vi "PCO_CamLinkSetImageParameters.vi"(8 "error in (no error)":errorcluster {"code" format="%x"}, 9 "wYres":u16, 10 "wXres":u16, 11 "ph":u64) -> (0 "error out":errorcluster {"code" format="%x"}, 2 "ErrorMessage":i32 format="%x", 3 "ph out":u64)   [LabVIEW 2019, in "SDK.lvlib" / "SpecialCommandsEdge.lvlib"]
doc: "Sets the parameters for an image transfer. Required for CameraLink interface, and recommended for other interface types. Call this function when there is a change in the effective image size through ROI os binning, or switching to RAM segment (cameras with internal memory) where the image size differs from the current segment."
uses:
  SpecialCommandsEdge.lvlib
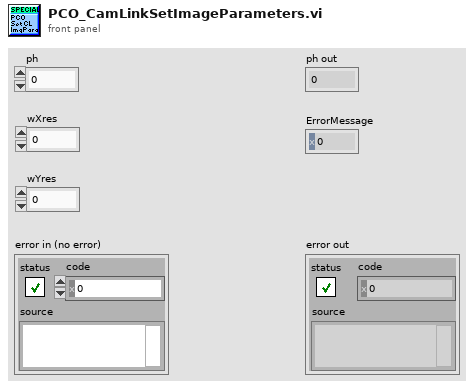
[diagram p1: front panel]
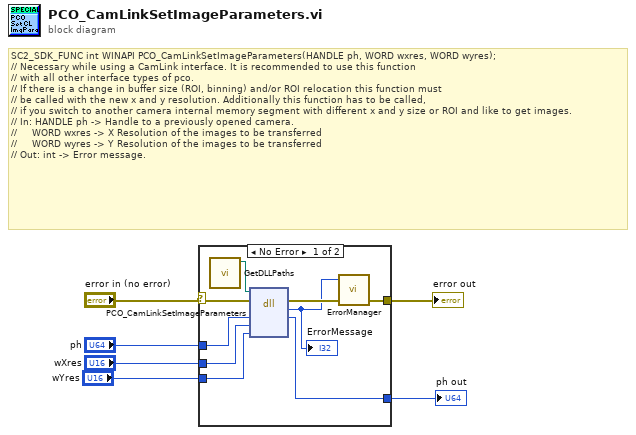
[diagram p0: block diagram]
diagram:
  # "SC2_SDK_FUNC int WINAPI PCO_CamLinkSetImageParameters(HANDLE ph, WORD wxres, WORD wyres);\n// Necessary while using a CamLink interface. It is recommended to use this function\n// with all other interface types of pco.\n// If there is a change in buffer size (ROI, binning) and/or ROI relocation this function must\n// be called with the new x and y resolution. Additionally this function has to be called,\n// if you switch to another camera internal memory segment with different x and y size or ROI and like to get images.\n// In: HANDLE ph -> Handle to a previously opened camera.\n//     WORD wxres -> X Resolution of the images to be transferred\n//     WORD wyres -> Y Resolution of the images to be transferred\n// Out: int -> Error message."
  n1 = case shown="No Error" "error in (no error)" {
    selector: "error in (no error)" -> [w13 w17]
    tunnel: "ph" -> [w15 w16]
    tunnel: [w14 w16] -> w5
    tunnel: [w11 w17] -> w4
    tunnel: "wXres" -> [w8 _]
    tunnel: "wYres" -> [w7 _]
    frame No Error {
      n2 = call "GetDLLPaths.vi"() -> ("SC2_Cam_Path"=w9:path)  [unwired: 8 in, 3 out]
      n3 = dll-call lib="?" fn="PCO_CamLinkSetImageParameters"(path in=w9, error in=w13, "ph"=w15, "wXres"=w8, "wYres"=w7) -> (error out=w12:errorcluster, "return type"=w10:i32, "ph"=w14:u64)  [unwired: 3 in, 1 out]
      "ErrorMessage" <- w10
      n4 = call "ErrorManager.vi"("error in (no error)"=w12, "error code"=w10) -> ("error out"=w11:errorcluster)  [unwired: 2 in, 1 out]
    }
    frame Error {
    }
  }
  "ph out" <- w5
  "error out" <- w4
